vi "FPGA_single_loop.vi"() -> ()   [LabVIEW 2015]
uses:
  <vilib>/rvi/Emulation/niFpgaGetClockAttributes.vi
  <vilib>/rvi/Emulation/niFpgaSctlEmulationGetInTimedLoop.vi
  <vilib>/rvi/Emulation/niFpgaEmulationReportErrorSimple.vi
  <vilib>/rvi/eio/common/nirviEmuTemplateMethod_errors.vi
  <vilib>/rvi/interface/RandomDataEmulation/nirviRandomDataMultiElementFPGAFIFO.vi
  <instcachedir>/0/nirviRandomDataMultiElementFPGAFIFO_8F99493546E24284B0D6A8E519C457F7.lvgen/nirviRandomDataMultiElementFPGAFIFO_8F99493546E24284B0D6A8E519C457F7_000.vi
  <vilib>/rvi/interface/RandomDataEmulation/niFpgaRandomDataHandleErrors.vi
  <vilib>/rvi/Emulation/niFpgaCriticalErrorInLSC.vi
  <vilib>/eio/EIONode/EIONode.xnode
  <vilib>/rvi/DataTransferAndStorage/Container/XNode/niFpgaContainer.xnode
  <vilib>/rvi/interface/RandomDataEmulation/nirviRandomDataFpgaMultiElementTemplate.vi
panel:
  out "Laser Loop Timer":u32
  in  "Laser J8":u16
  in  "Laser J5":u16
  in  "Laser J4":u16
  in  "Laser J1":u16
  in  "stop Laser":bool
  in  "LED switch-2 J8":bool
  in  "LED switch-1 J8":bool
  in  "Low Period (ticks) J8":u32=40000000
  in  "LED intensity J8":u32=40000000
  in  "LED switch-2 J5":bool
  in  "LED switch-1 J5":bool
  in  "Low Period (ticks) J5":u32=40000000
  in  "LED intensity J5":u32=40000000
  in  "LED switch-2 J4":bool
  in  "LED switch-1 J4":bool
  in  "Low Period (ticks) J4":u32=40000000
  in  "LED intensity J4":u32=40000000
  in  "stop LED":bool
  in  "Low Period (ticks) J1":u32=40000000
  in  "LED intensity J1":u32=40000000
  in  "LED switch-1 J1":bool
  in  "LED switch-2 J1":bool
  out "LED loop time":u32
  in  "FPGA Stop":bool
  out "Frame Count":i16=5
  in  "IRQ Bit (0-31)":u8
  in  "Wait Until IRQ Cleared?":bool
  out "Timed Out?":bool
  in  "double number of samples to take per frame":u16=1540
  in  "Half-clocks between frames":u16=1600
  out "Sensor Loop Time":u32
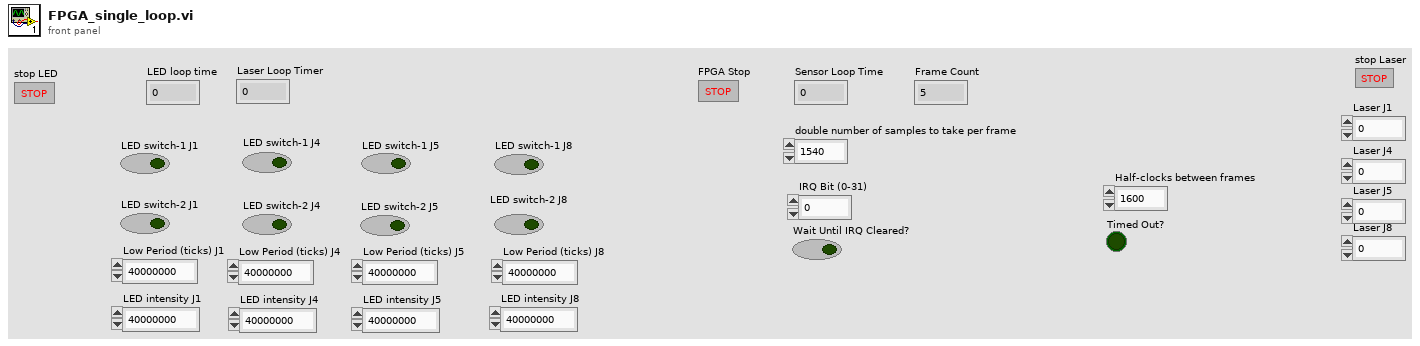
[diagram p1: front panel]
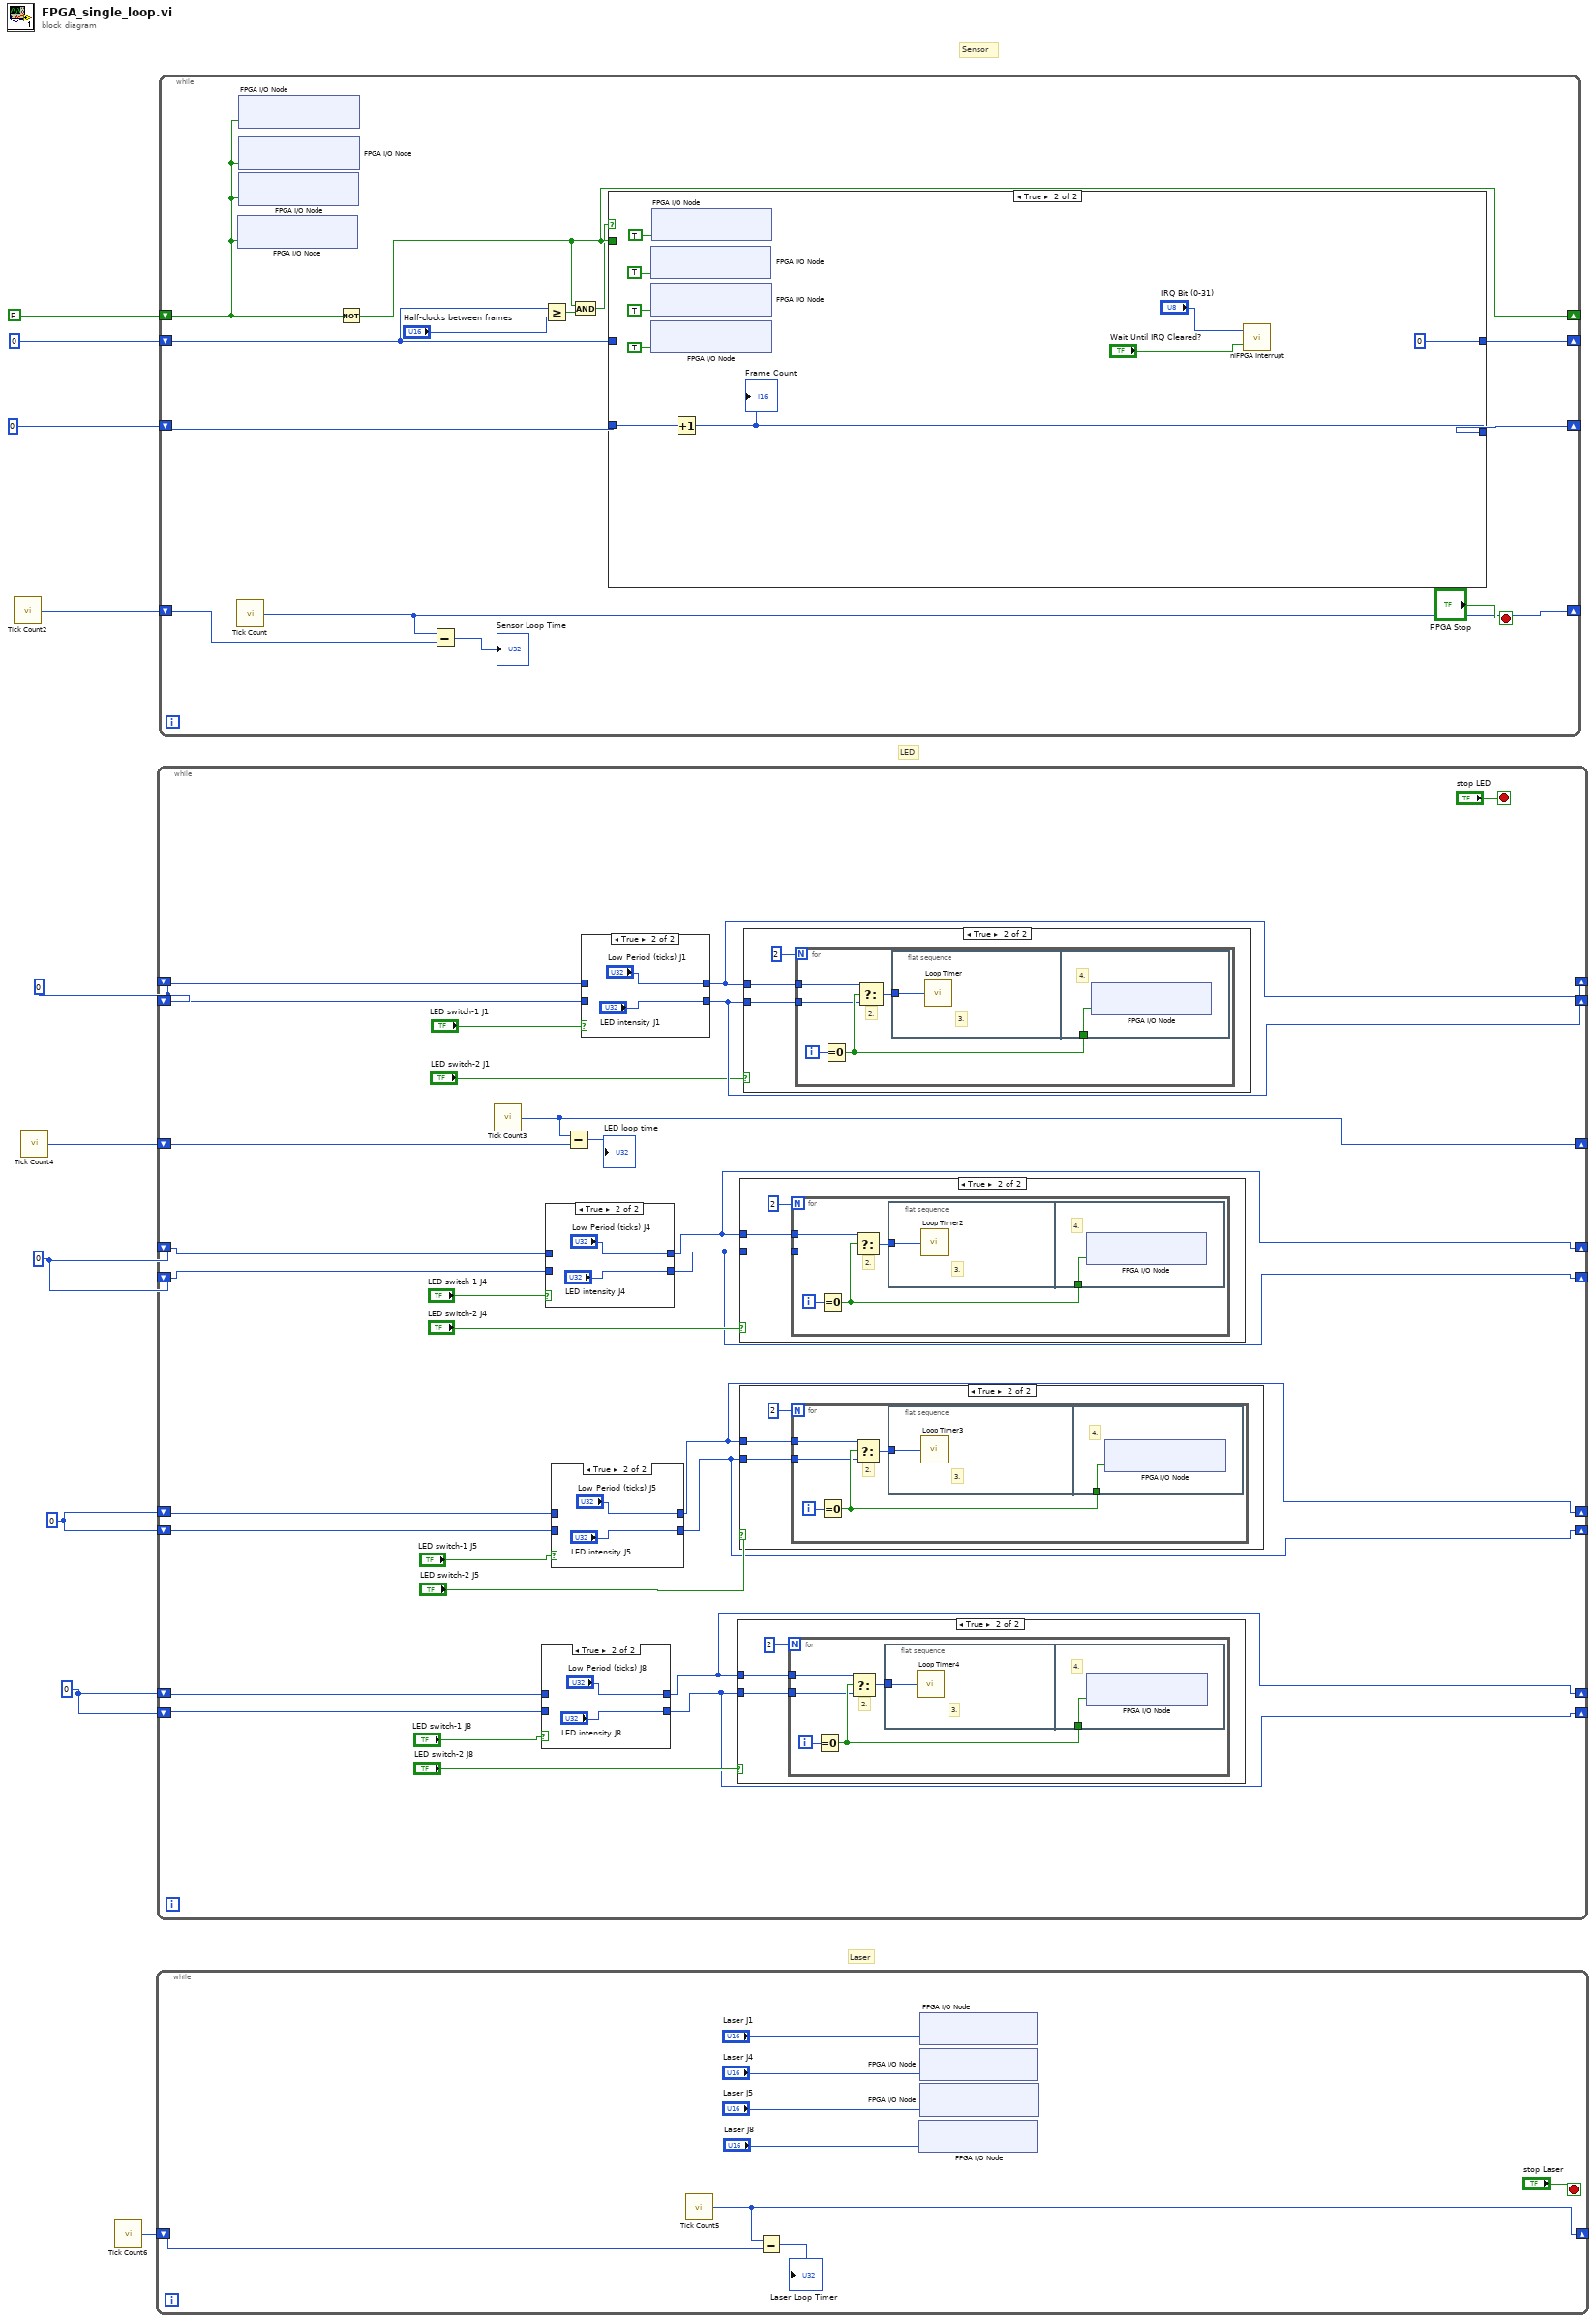
[diagram p0: block diagram]
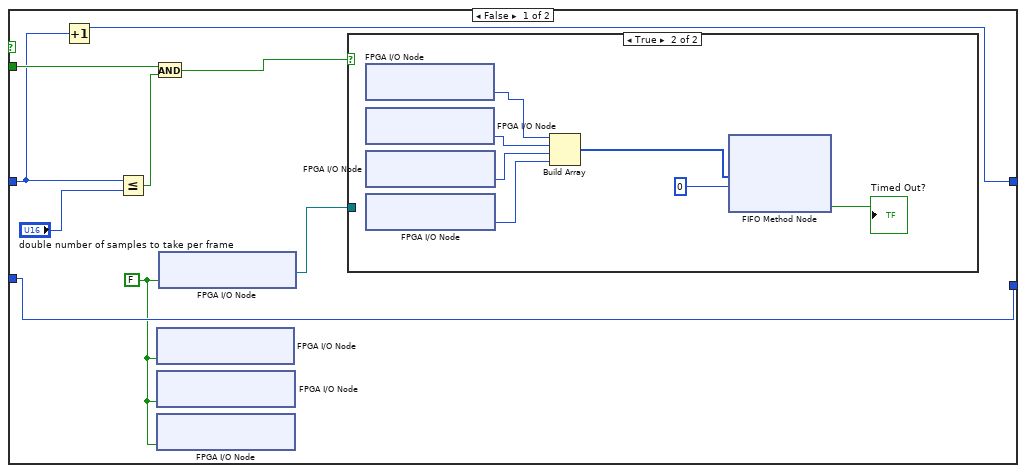
[diagram p10: hidden frame]
diagram:
  w2 = u32 0 ("High Period")
  w3 = u32 0 ("High Period")
  w4 = u32 0 ("High Period")
  w6 = u32 0 ("High Period")
  # "Laser"
  # "LED"
  # "Sensor"
  n1 = call "Tick Count2"() -> ("Tick Count(Ticks)"=w7:u32)
  n2 = call "Tick Count4"() -> ("Tick Count(Ticks)"=w5:u32)
  n3 = call "Tick Count6"() -> ("Tick Count(Ticks)"=w1:u32)
  n4 = while {
    shift-right: [w11] -> _
    shift-left: w1 -> [w12]
    stop <- "stop Laser" stop-if-true
    n5 = call "Tick Count5"() -> ("Tick Count(Ticks)"=w11:u32)
    n6 = Subtract(x=w11, y=w12) -> (x-y=→"Laser Loop Timer":u32)
    n7 = xnode "FPGA I/O Node"("ConnectorA/AO1"="Laser J8") -> ()  [unwired: 1 in, 1 out]
    n8 = xnode "FPGA I/O Node"("ConnectorB/AO0"="Laser J1") -> ()  [unwired: 1 in, 1 out]
    n9 = xnode "FPGA I/O Node"("ConnectorB/AO1"="Laser J4") -> ()  [unwired: 1 in, 1 out]
    n10 = xnode "FPGA I/O Node"("ConnectorA/AO0"="Laser J5") -> ()  [unwired: 1 in, 1 out]
  }
  n11 = while {
    shift-right: [w41] -> _
    shift-left: w6 -> [w45]
    shift-right: [w42] -> _
    shift-left: w6 -> [w44]
    shift-right: [w39] -> _
    shift-left: w5 -> [w38]
    shift-right: [w32] -> _
    shift-left: w4 -> [w34]
    shift-right: [w31] -> _
    shift-left: w4 -> [w33]
    shift-right: [w26] -> _
    shift-left: w3 -> [w28]
    shift-right: [w25] -> _
    shift-left: w3 -> [w27]
    shift-right: [w20] -> _
    shift-left: w2 -> [w22]
    shift-right: [w19] -> _
    shift-left: w2 -> [w21]
    stop <- "stop LED" stop-if-true
    n12 = call "Tick Count3"() -> ("Tick Count(Ticks)"=w39:u32)
    n13 = case shown="True" "LED switch-1 J8" {
      tunnel: [w58 "Low Period (ticks) J8"] -> w20
      tunnel: [w57 "LED intensity J8"] -> w19
      tunnel: w22 -> [w58 _]
      tunnel: w21 -> [w57 _]
      frame False {
      }
      frame True {
      }
    }
    n14 = case shown="True" "LED switch-1 J4" {
      tunnel: [w86 "Low Period (ticks) J4"] -> w32
      tunnel: [w85 "LED intensity J4"] -> w31
      tunnel: w34 -> [w86 _]
      tunnel: w33 -> [w85 _]
      frame False {
      }
      frame True {
      }
    }
    n15 = case shown="True" "LED switch-1 J5" {
      tunnel: [w72 "Low Period (ticks) J5"] -> w26
      tunnel: [w71 "LED intensity J5"] -> w25
      tunnel: w28 -> [w72 _]
      tunnel: w27 -> [w71 _]
      frame False {
      }
      frame True {
      }
    }
    n16 = Subtract(x=w39, y=w38) -> (x-y=→"LED loop time":u32)
    n17 = case shown="True" "LED switch-1 J1" {
      tunnel: [w100 "Low Period (ticks) J1"] -> w41
      tunnel: [w99 "LED intensity J1"] -> w42
      tunnel: w45 -> [w100 _]
      tunnel: w44 -> [w99 _]
      frame False {
      }
      frame True {
      }
    }
    n18 = case shown="True" "LED switch-2 J8" {
      tunnel: w20 -> [_ w48]
      tunnel: w19 -> [_ w47]
      frame False {
      }
      frame True {
        n19 = for {
          N: 2 -> [_]
          tunnel: w48 -> [w51]
          tunnel: w47 -> [w50]
          i -> [w53]
          # "2."
          n20 = Equal To 0?(x=w53) -> (x = 0?=w52:bool)
          n21 = Select(t=w51, s=w52, f=w50) -> (s? t:f=w54:u32)
          n22 = flat-sequence {
            tunnel: w54 -> [w55]
            tunnel: w52 -> [w56]
            frame #0 {
              # "3."
              n23 = call "Loop Timer4"("Count(Ticks)"=w55) -> ()  [unwired: 1 out]
            }
            frame #1 {
              # "4."
              n24 = xnode "FPGA I/O Node"("ConnectorA/DIO9"=w56) -> ()  [unwired: 1 in, 1 out]
            }
          }
        }
      }
    }
    n25 = case shown="True" "LED switch-2 J4" {
      tunnel: w32 -> [_ w76]
      tunnel: w31 -> [_ w75]
      frame False {
      }
      frame True {
        n26 = for {
          N: 2 -> [_]
          tunnel: w76 -> [w79]
          tunnel: w75 -> [w78]
          i -> [w81]
          # "2."
          n27 = Equal To 0?(x=w81) -> (x = 0?=w80:bool)
          n28 = Select(t=w79, s=w80, f=w78) -> (s? t:f=w82:u32)
          n29 = flat-sequence {
            tunnel: w82 -> [w83]
            tunnel: w80 -> [w84]
            frame #0 {
              # "3."
              n30 = call "Loop Timer2"("Count(Ticks)"=w83) -> ()  [unwired: 1 out]
            }
            frame #1 {
              # "4."
              n31 = xnode "FPGA I/O Node"("ConnectorB/DIO9"=w84) -> ()  [unwired: 1 in, 1 out]
            }
          }
        }
      }
    }
    n32 = case shown="True" "LED switch-2 J5" {
      tunnel: w26 -> [_ w62]
      tunnel: w25 -> [_ w61]
      frame False {
      }
      frame True {
        n33 = for {
          N: 2 -> [_]
          tunnel: w62 -> [w65]
          tunnel: w61 -> [w64]
          i -> [w67]
          # "2."
          n34 = Equal To 0?(x=w67) -> (x = 0?=w66:bool)
          n35 = Select(t=w65, s=w66, f=w64) -> (s? t:f=w68:u32)
          n36 = flat-sequence {
            tunnel: w68 -> [w69]
            tunnel: w66 -> [w70]
            frame #0 {
              # "3."
              n37 = call "Loop Timer3"("Count(Ticks)"=w69) -> ()  [unwired: 1 out]
            }
            frame #1 {
              # "4."
              n38 = xnode "FPGA I/O Node"("ConnectorA/DIO8"=w70) -> ()  [unwired: 1 in, 1 out]
            }
          }
        }
      }
    }
    n39 = case shown="True" "LED switch-2 J1" {
      tunnel: w41 -> [_ w90]
      tunnel: w42 -> [_ w89]
      frame False {
      }
      frame True {
        n40 = for {
          N: 2 -> [_]
          tunnel: w90 -> [w93]
          tunnel: w89 -> [w92]
          i -> [w95]
          # "2."
          n41 = Equal To 0?(x=w95) -> (x = 0?=w94:bool)
          n42 = Select(t=w93, s=w94, f=w92) -> (s? t:f=w96:u32)
          n43 = flat-sequence {
            tunnel: w96 -> [w97]
            tunnel: w94 -> [w98]
            frame #0 {
              # "3."
              n44 = call "Loop Timer"("Count(Ticks)"=w97) -> ()  [unwired: 1 out]
            }
            frame #1 {
              # "4."
              n45 = xnode "FPGA I/O Node"("ConnectorB/DIO8"=w98) -> ()  [unwired: 1 in, 1 out]
            }
          }
        }
      }
    }
  }
  n46 = while {
    shift-right: [w115] -> _
    shift-left: FALSE ("ConnectorB/DIO0") -> [w103]
    shift-right: [w112] -> _
    shift-left: u16 0 -> [w114]
    shift-right: [w110] -> _
    shift-left: i16 0 -> [w111]
    shift-right: [w106] -> _
    shift-left: w7 -> [w105]
    stop <- "FPGA Stop" stop-if-true
    n47 = call "Tick Count"() -> ("Tick Count(Ticks)"=w106:u32)
    n48 = xnode "FPGA I/O Node"("ConnectorB/DIO0"=w103) -> ()  [unwired: 1 in, 1 out]
    n49 = xnode "FPGA I/O Node"("ConnectorA/DIO0"=w103) -> ()  [unwired: 1 in, 1 out]
    n50 = xnode "FPGA I/O Node"("ConnectorA/DIO2"=w103) -> ()  [unwired: 1 in, 1 out]
    n51 = xnode "FPGA I/O Node"("ConnectorB/DIO2"=w103) -> ()  [unwired: 1 in, 1 out]
    n52 = Not(x=w103) -> (.not. x?=w115:bool)
    n53 = Subtract(x=w106, y=w105) -> (x-y=→"Sensor Loop Time":u32)
    n54 = Greater Or Equal?(x=w114, y="Half-clocks between frames") -> (x >= y?=w109:bool)
    n55 = And(x=w115, y=w109) -> (x .and. y?=w107:bool)
    n56 = case shown="True" w107 {
      tunnel: w114 -> [w120 _]
      tunnel: [w118 u16 0] -> w112
      tunnel: w115 -> [w124 _]
      tunnel: w111 -> [w119 w138]
      tunnel: [w119 w137] -> w110
      frame False {
        w116 = FALSE ("ConnectorB/DIO1")
        n57 = Increment(x=w120) -> (x+1=w118:u16)
        n58 = Less Or Equal?(x=w120, y="double number of samples to take per frame") -> (x <= y?=w122:bool)
        n59 = And(x=w124, y=w122) -> (x .and. y?=w123:bool)
        n60 = xnode "FPGA I/O Node"("ConnectorB/DIO3"=w116) -> ()  [unwired: 1 in, 1 out]
        n61 = xnode "FPGA I/O Node"("ConnectorA/DIO1"=w116) -> ()  [unwired: 1 in, 1 out]
        n62 = xnode "FPGA I/O Node"("ConnectorA/DIO3"=w116) -> ()  [unwired: 1 in, 1 out]
        n63 = xnode "FPGA I/O Node"("ConnectorB/DIO1"=w116) -> ("FPGA I/O Out"=w121:refnum<k21>)  [unwired: 1 in]
        n64 = case shown="True" w123 {
          tunnel: w121 -> [_ _]
          frame False {
          }
          frame True {
            n65 = xnode "FPGA I/O Node"() -> ("ConnectorB/AI0"=w128:u16)  [unwired: 1 in, 1 out]
            n66 = xnode "FPGA I/O Node"() -> ("ConnectorB/AI1"=w127:u16)  [unwired: 1 in, 1 out]
            n67 = xnode "FPGA I/O Node"() -> ("ConnectorA/AI0"=w126:u16)  [unwired: 1 in, 1 out]
            n68 = xnode "FPGA I/O Node"() -> ("ConnectorA/AI1"=w125:u16)  [unwired: 1 in, 1 out]
            n69 = Build Array(w128, w127, w126, w125) -> (w129:u16[])
            n70 = xnode ("FIFO Method Node")("Element"=w129, "Timeout"=0) -> ("Timed Out?"=→"Timed Out?":bool)  [unwired: 1 in, 1 out]
          }
        }
      }
      frame True {
        n71 = xnode "FPGA I/O Node"("ConnectorB/DIO3"=TRUE ("ConnectorB/DIO1")) -> ()  [unwired: 1 in, 1 out]
        n72 = xnode "FPGA I/O Node"("ConnectorA/DIO1"=TRUE ("ConnectorB/DIO1")) -> ()  [unwired: 1 in, 1 out]
        n73 = xnode "FPGA I/O Node"("ConnectorA/DIO3"=TRUE ("ConnectorB/DIO1")) -> ()  [unwired: 1 in, 1 out]
        n74 = xnode "FPGA I/O Node"("ConnectorB/DIO1"=TRUE) -> ()  [unwired: 1 in, 1 out]
        n75 = Increment(x=w138) -> (x+1=w137:i16)
        "Frame Count" <- w137
        n76 = call <vilib>:"niFPGA Interrupt.vi"("Wait Until Cleared (F)"="Wait Until IRQ Cleared?", "IRQ Number (0)"="IRQ Bit (0-31)") -> ()  [unwired: 1 in]
      }
    }
  }
